vi "Excel Create Printable Sheet.vi"(0 "Sheets Ref In":refnum<k7>, 1 "RowsFirstHeader":i32, 2 "RowsHeadersAfter":i32, 5 "Stat Array":string[][](array[string]), 7 "CMD Step":dbl format="%#_13g", 9 "HeaderInfo":string[](array[string]), 11 "Error In":errorcluster, 12 "RowsFirstPage":i32, 13 "RowsPagesAfter":i32) -> (4 "Sheets Ref Out":refnum<k7>, 15 "Error Out":errorcluster)   [LabVIEW 2013]
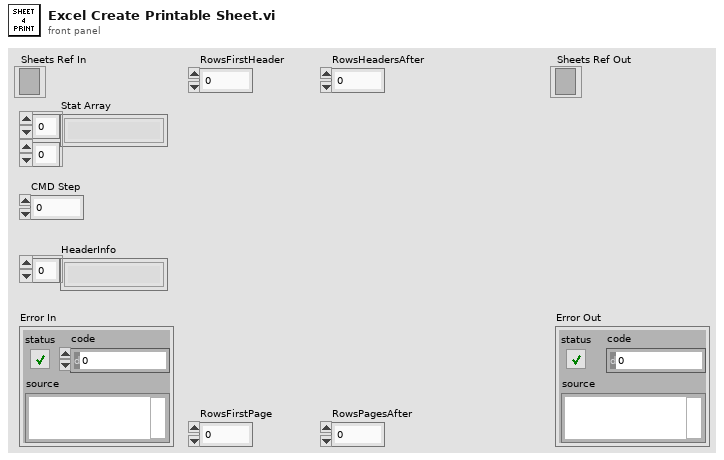
[diagram p1: front panel]
types:
  T1 = cluster{"StartData":i32, "SectionLength":i32, "Have2Split":bool}
  T2 = cluster{"PageStartingIndex":i32, "PageLength":i32}[]
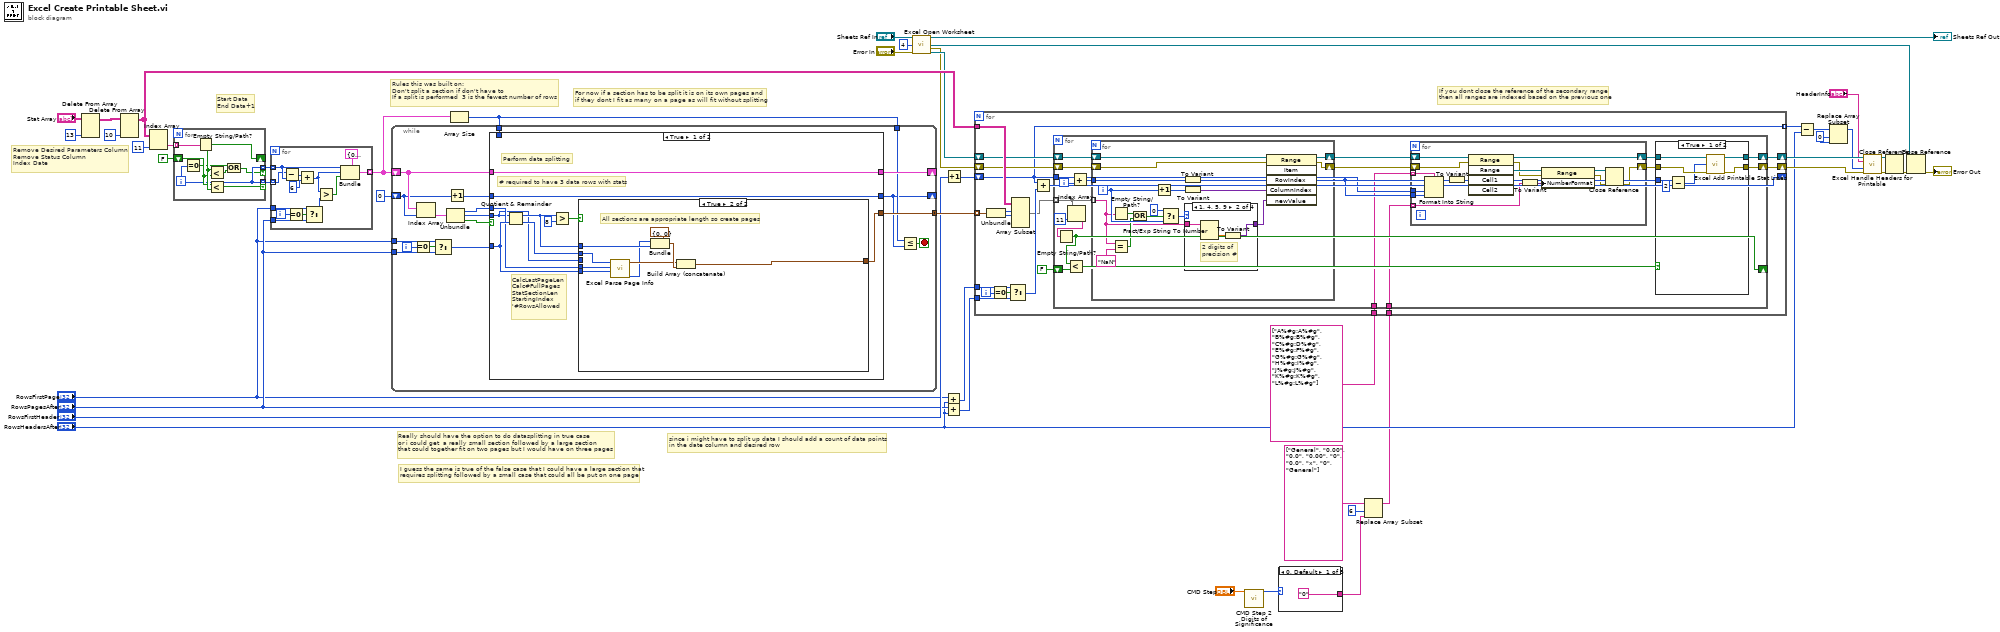
[diagram p0: block diagram]
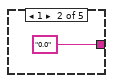
[diagram p2: hidden frame]
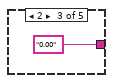
[diagram p3: hidden frame]
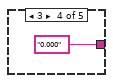
[diagram p4: hidden frame]
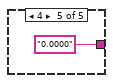
[diagram p5: hidden frame]
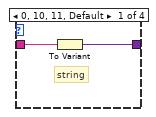
[diagram p7: hidden frame]
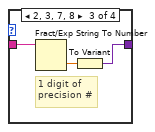
[diagram p8: hidden frame]
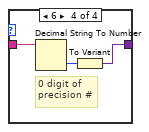
[diagram p9: hidden frame]
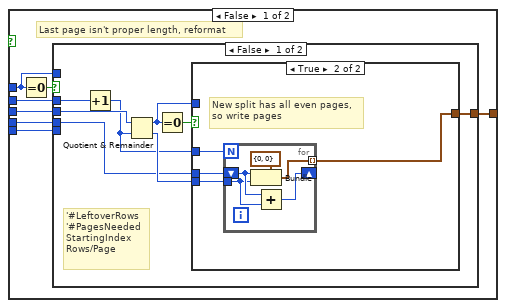
[diagram p10: hidden frame]
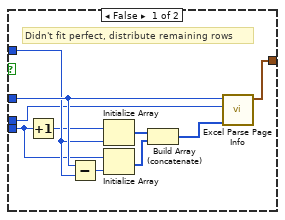
[diagram p11: hidden frame]
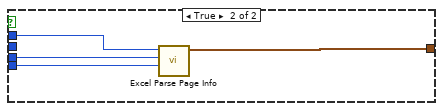
[diagram p12: hidden frame]
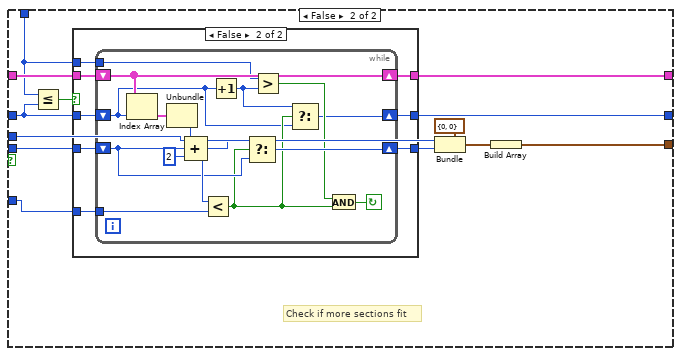
[diagram p13: hidden frame]
diagram:
  w31 = 0 ("index")
  # "If you dont close the reference of the secondary range\nthen all ranges are indexed based on the previous one"
  # "Rules this was built on:\nDon't split a section if don't have to\nIf a split is performed  3 is the fewest number of rows"
  # "For now if a section has to be split it is on its own pages and\nif they dont I fit as many on a page as will fit without splitting"
  # "since i might have to split up data I should add a count of data points\nin the date column and desired row"
  # "I guess the same is true of the false case that I could have a large section that\nrequires splitting followed by a small case that could all be put on one page"
  # "Really should have the option to do datasplitting in true case\nor i could get  a really small section followed by a large section\nthat could together fit on two pages but I would have on three pages"
  # "Start Data\nEnd Data+1"
  # "Remove Desired Parameters Column\nRemove Status Column\nIndex Date"
  n1 = Delete From Array(array="Stat Array", index (col)=13 ("disabled index (col)")) -> (array with subset deleted=w45:string[][])  [unwired: 2 in, 1 out]
  n2 = Delete From Array(array=w45, index (col)=10 ("disabled index (col)")) -> (array with subset deleted=w34:string[][])  [unwired: 2 in, 1 out]
  n3 = Index Array(array=w34, index (col)=11 ("disabled index (col)")) -> (element=w41:string[])  [unwired: 1 in]
  n4 = for {
    tunnel: w41 -> [w54] mode=indexing
    shift-right: [w53] -> _
    shift-left: FALSE -> [w52]
    tunnel: [w50] -> w39 mode=indexing if=w49
    tunnel: [w50] -> w38 mode=indexing if=w51
    i -> [w50]
    n5 = Equal To 0?(x=w50) -> (x = 0?=w47:bool)
    n6 = Empty String/Path?(string/path=w54) -> (empty?=w53:bool)
    n7 = Less?(x=w53, y=w52) -> (x < y?=w48:bool)
    n8 = Less?(x=w52, y=w53) -> (x < y?=w51:bool)
    n9 = Or(x=w47, y=w48) -> (x .or. y?=w49:bool)
  }
  n10 = for {
    tunnel: w39 -> [w67] mode=indexing
    tunnel: w38 -> [w66] mode=indexing
    tunnel: [w65] -> w36 mode=indexing
    tunnel: "RowsFirstPage" -> [w59]
    tunnel: "RowsPagesAfter" -> [w58]
    i -> [w60]
    n11 = Subtract(x=w66, y=w67) -> (x-y=w64:i32)
    n12 = Equal To 0?(x=w60) -> (x = 0?=w61:bool)
    n13 = Add(x=w64, y=6) -> (x+y=w57:i32)
    n14 = Select(t=w59, s=w61, f=w58) -> (s? t:f=w56:i32)
    n15 = Greater?(x=w57, y=w56) -> (0:w55:bool)
    n16 = Bundle(cluster=T1 {"StartData"=0, "SectionLength"=0, "Have2Split"=FALSE}, "StartData"=w67, "SectionLength"=w57, "Have2Split"=w55) -> (w65:T1)
  }
  n17 = Array Size(array=w36) -> (size(s)=w13:i32)
  n18 = while {
    tunnel: "RowsFirstPage" -> [w85]
    tunnel: "RowsPagesAfter" -> [w84]
    shift-right: [w83] -> _
    shift-left: w36 -> [w70]
    shift-right: [w73] -> _
    shift-left: 0 -> [w69]
    tunnel: w13 -> [w74]
    tunnel: [w75] -> w35 mode=concatenating
    tunnel: w13 -> [w71]
    i -> [w77]
    stop <- w72 stop-if-true
    n19 = Equal To 0?(x=w77) -> (x = 0?=w78:bool)
    n20 = Index Array(array=w70, index=w69) -> (element=w68:T1)
    n21 = Select(t=w85, s=w78, f=w84) -> (s? t:f=w79:i32)
    n22 = Unbundle(w68) -> ("StartData"=w82:i32, "SectionLength"=w81:i32, "Have2Split"=w76:bool)
    n23 = Increment(x=w69) -> (x+1=w80:i32)
    n24 = case shown="True" w76 {
      tunnel: w70 -> [w95 w155]
      tunnel: [w95 w154] -> w83
      tunnel: w82 -> [w89 w150]
      tunnel: w81 -> [w86 w153]
      tunnel: w80 -> [w94 w144]
      tunnel: [w87 w147] -> w75
      tunnel: [w94 w146] -> w73
      tunnel: w79 -> [w90 w152]
      tunnel: w71 -> [_ w145]
      frame True {
        # "CalcLastPageLen\nCalc#FullPages\nStatSectionLen\nStartingIndex\n'#RowsAllowed"
        # "# required to have 3 data rows with stats"
        # "Perform data splitting"
        n25 = Quotient & Remainder(x=w86, y=w90) -> (x-y*floor(x/y)=w88:i32, floor(x/y)=w91:i32)
        n26 = Greater?(x=w88, y=8) -> (0:w92:bool)
        n27 = case shown="True" w92 {
          tunnel: w91 -> [w99 w138]
          tunnel: w90 -> [w100 w137]
          tunnel: w89 -> [w101 w135]
          tunnel: w88 -> [w97 w141]
          tunnel: [w98 w139] -> w87
          tunnel: w86 -> [w96 _]
          frame False {
            # "Last page isn't proper length, reformat"
            n28 = Equal To 0?(x=w97) -> (x = 0?=w102:bool)
            n29 = case shown="False" w102 {
              tunnel: w101 -> [w108 w131]
              tunnel: w100 -> [_ w132]
              tunnel: w99 -> [w103 w130]
              tunnel: [w106 w133] -> w98
              tunnel: w97 -> [_ _]
              tunnel: w96 -> [w107 _]
              frame False {
                # "'#LeftoverRows\n'#PagesNeeded\nStartingIndex\nRows/Page"
                n30 = Increment(x=w103) -> (x+1=w104:i32)
                n31 = Quotient & Remainder(x=w107, y=w104) -> (x-y*floor(x/y)=w105:i32, floor(x/y)=w109:i32)
                n32 = Equal To 0?(x=w105) -> (x = 0?=w110:bool)
                n33 = case shown="True" w110 {
                  tunnel: w109 -> [w115 w124]
                  tunnel: w108 -> [w111 w123]
                  tunnel: [w120 w122] -> w106
                  tunnel: w105 -> [w118 _]
                  tunnel: w104 -> [w119 w121]
                  frame False {
                    # "Didn't fit perfect, distribute remaining rows"
                    n34 = Increment(x=w115) -> (x+1=w116:i32)
                    n35 = Subtract(x=w119, y=w118) -> (x-y=w117:i32)
                    n36 = Initialize Array(w116, w118) -> (w114:i32[])
                    n37 = Initialize Array(w115, w117) -> (w113:i32[])
                    n38 = Build Array (concatenate)(w114, w113) -> (w112:i32[])
                    n39 = call "Excel Parse Page Info.vi"("[PageLengths]"=w112, "StartingIndex"=w111, "# of Pages"=w119) -> ("Page Info"=w120:T2)  [unwired: 7 in, 1 out]
                  }
                  frame True {
                    # "New split has all even pages,\nso write pages"
                    n40 = for {
                      N: w121 -> [_]
                      tunnel: w124 -> [w126]
                      shift-right: [w125] -> _
                      shift-left: w123 -> [w127]
                      tunnel: [w128] -> w122 mode=indexing
                      n41 = Bundle(cluster=cluster{"StartPage":i32, "PageLength":i32} {"StartPage"=0, "PageLength"=0}, "StartPage"=w127, "PageLength"=w126) -> (w128:cluster{"StartPage":i32, "PageLength":i32})
                      n42 = Add(x=w127, y=w126) -> (x+y=w125:i32)
                    }
                  }
                }
              }
              frame True {
                n43 = call "Excel Parse Page Info.vi"("PageLength"=w132, "StartingIndex"=w131, "# of Pages"=w130) -> ("Page Info"=w133:T2)  [unwired: 7 in, 1 out]
              }
            }
          }
          frame True {
            # "All sections are appropriate length so create pages"
            n44 = call "Excel Parse Page Info.vi"("PageLength"=w137, "StartingIndex"=w135, "# of Pages"=w138) -> ("IndexOut"=w134:i32, "Page Info"=w136:T2)  [unwired: 7 in]
            n45 = Bundle(cluster=cluster{"StartPage":i32, "PageLength":i32} {"StartPage"=0, "PageLength"=0}, "StartPage"=w134, "PageLength"=w141) -> (w140:cluster{"StartPage":i32, "PageLength":i32})
            n46 = Build Array (concatenate)(w136, w140) -> (w139:cluster{"StartPage":i32, "PageLength":i32}[])
          }
        }
      }
      frame False {
        # "Check if more sections fit"
        n47 = Less Or Equal?(x=w145, y=w144) -> (x <= y?=w143:bool)
        n48 = case shown="False" w143 {
          tunnel: w155 -> [w158 w166]
          tunnel: [w158 w165] -> w154
          tunnel: w153 -> [w156 w164]
          tunnel: w144 -> [w157 w163]
          tunnel: w152 -> [_ w162]
          tunnel: [w156 w161] -> w149
          tunnel: [w157 w160] -> w146
          tunnel: w145 -> [_ w159]
          frame True {
          }
          frame False {
            n49 = while {
              shift-right: [w181] -> w165
              shift-left: w166 -> [w181]
              shift-right: [w174] -> w161
              shift-left: w164 -> [w175]
              tunnel: w162 -> [w177]
              shift-right: [w168] -> w160
              shift-left: w163 -> [w169]
              tunnel: w159 -> [w167]
              stop <- w173 continue-if-true
              n50 = Index Array(array=w181, index=w169) -> (element=w180:T1)
              n51 = Unbundle(w180) -> ("SectionLength"=w179:i32)  [unwired: 2 out]
              n52 = Compound Arithmetic op=ADD(w179, w175, 2 ("value")) -> (w176:i32)
              n53 = Less?(x=w176, y=w177) -> (x < y?=w171:bool)
              n54 = Increment(x=w169) -> (x+1=w170:i32)
              n55 = Select(t=w176, s=w171, f=w175) -> (s? t:f=w174:i32)
              n56 = Greater?(x=w167, y=w170) -> (0:w172:bool)
              n57 = Select(t=w170, s=w171, f=w169) -> (s? t:f=w168:i32)
              n58 = And(x=w172, y=w171) -> (x .and. y?=w173:bool)
            }
          }
        }
        n59 = Bundle(cluster=cluster{"StartPage":i32, "PageLength":i32} {"StartPage"=0, "PageLength"=0}, "StartPage"=w150, "PageLength"=w149) -> (w148:cluster{"StartPage":i32, "PageLength":i32})
        n60 = Build Array(w148) -> (w147:cluster{"StartPage":i32, "PageLength":i32}[])
      }
    }
    n61 = Less Or Equal?(x=w74, y=w73) -> (x <= y?=w72:bool)
  }
  n62 = call "Excel Open Worksheet.vi"("Sheets Ref In"="Sheets Ref In", "Sheet#"=4, "Error In"="Error In") -> ("Sheets Ref Out"=→"Sheets Ref Out":refnum<k7>, "Worksheet Ref Out"=w21:refnum<k7>, "Error Out"=w28:errorcluster, "Cells Ref Out"=w29:refnum<k7>)  [unwired: 9 in]
  n63 = Add(x="RowsFirstPage", y="RowsHeadersAfter") -> (x+y=w8:i32)
  n64 = Add(x="RowsPagesAfter", y="RowsHeadersAfter") -> (x+y=w11:i32)
  n65 = Increment(x="RowsFirstHeader") -> (x+1=w14:i32)
  n66 = call "CMD Step 2 Digits of Significance.vi"("CMD Step"="CMD Step") -> ("Digits of Significance"=w5:i32)  [unwired: 14 in]
  n67 = case shown="0, Default" w5 {
    tunnel: ["0" "0.0" "0.00" "0.000" "0.0000"] -> w7
    frame 0, Default {
    }
    frame 1 {
    }
    frame 2 {
    }
    frame 3 {
    }
    frame 4 {
    }
  }
  n68 = Replace Array Subset(array=string[] ["General", "0.00", "0.0", "0.00", "0", "0.0", "x", "0", "General"], new element=w7, index=6) -> (w1:string[])
  n69 = for {
    tunnel: w35 -> [w205] mode=indexing
    tunnel: w34 -> [w204]
    shift-right: [w191] -> w27
    shift-left: w29 -> [w201]
    shift-right: [w192] -> w26
    shift-left: w28 -> [w200]
    shift-right: [w196] -> _
    shift-left: w14 -> [w190]
    tunnel: w11 -> [w195]
    tunnel: w8 -> [w194]
    tunnel: [w190] -> w33 mode=indexing
    tunnel: string[] ["A%#g:A%#g", "B%#g:B%#g", "C%#g:D%#g", "E%#g:F%#g", "G%#g:G%#g", "H%#g:I%#g", "J%#g:J%#g", "K%#g:K%#g", "L%#g:L%#g"] -> [w188]
    tunnel: w1 -> [w187]
    i -> [w198]
    n70 = Unbundle(w205) -> ("StartPage"=w203:i32, "PageLength"=w202:i32)
    n71 = Equal To 0?(x=w198) -> (x = 0?=w199:bool)
    n72 = Select(t=w194, s=w199, f=w195) -> (s? t:f=w197:i32)
    n73 = Array Subset(array=w204, index (row)=w203, length (row)=w202) -> (w193:string[][])  [unwired: 2 in]
    n74 = Add(x=w190, y=w197) -> (x+y=w196:i32)
    n75 = for {
      shift-right: [w214] -> w191
      shift-left: w201 -> [w224]
      shift-right: [w215] -> w192
      shift-left: w200 -> [w223]
      tunnel: w193 -> [w221] mode=indexing
      tunnel: w190 -> [w208]
      shift-right: [w218] -> _
      shift-left: FALSE -> [w217]
      tunnel: w188 -> [w207]
      tunnel: w187 -> [w206]
      i -> [w222]
      n76 = Index Array(array=w221, index=11) -> (element=w219:string)
      n77 = Empty String/Path?(string/path=w219) -> (empty?=w218:bool)
      n78 = Less?(x=w218, y=w217) -> (x < y?=w216:bool)
      n79 = Add(x=w208, y=w222) -> (x+y=w209:i32)
      n80 = for {
        shift-right: [w264] -> w213
        shift-left: w224 -> [w265]
        shift-right: [w263] -> w212
        shift-left: w223 -> [w262]
        tunnel: w221 -> [w251] mode=indexing
        tunnel: w209 -> [w254]
        i -> [w257]
        n81 = Empty String/Path?(string/path=w251) -> (empty?=w250:bool)
        n82 = Equal?(x=w251, y="NaN") -> (x = y?=w253:bool)
        n83 = Or(x=w250, y=w253) -> (x .or. y?=w249:bool)
        n84 = Increment(x=w257) -> (x+1=w259:i32)
        n85 = Select(t=0, s=w249, f=w257) -> (s? t:f=w255:i32)
        n86 = To Variant(anything=w254) -> (Variant=w261:variant)
        n87 = To Variant(anything=w259) -> (Variant=w260:variant)
        n88 = case shown="1, 4, 5, 9" w255 {
          tunnel: w251 -> [w267 w270 w273 w276]
          tunnel: [w266 w268 w271 w274] -> w258
          frame 0, 10, 11, Default {
            # "string"
            n89 = To Variant(anything=w267) -> (Variant=w266:variant)
          }
          frame 1, 4, 5, 9 {
            # "2 digits of\nprecision #"
            n90 = Fract/Exp String To Number(string=w270) -> (number=w269:dbl)  [unwired: 3 in, 1 out]
            n91 = To Variant(anything=w269) -> (Variant=w268:variant)
          }
          frame 2, 3, 7, 8 {
            # "1 digit of\nprecision #"
            n92 = Fract/Exp String To Number(string=w273) -> (number=w272:dbl)  [unwired: 3 in, 1 out]
            n93 = To Variant(anything=w272) -> (Variant=w271:variant)
          }
          frame 6 {
            # "0 digit of\nprecision #"
            n94 = Decimal String To Number(string=w276) -> (number=w275:i32)  [unwired: 2 in, 1 out]
            n95 = To Variant(anything=w275) -> (Variant=w274:variant)
          }
        }
        n96 = invoke class="Range" method="Item"(reference=w265, error in=w262, "RowIndex"=w261, "ColumnIndex"=w260, "newValue"=w258) -> (reference out=w264:refnum<k7>, error out=w263:errorcluster)  [unwired: 1 in, 4 out]
      }
      n97 = for {
        shift-right: [w227] -> w211
        shift-left: w213 -> [w233]
        shift-right: [w226] -> w210
        shift-left: w212 -> [w232]
        tunnel: w206 -> [w237] mode=indexing
        tunnel: w207 -> [w236] mode=indexing
        tunnel: w208 -> [w235]
        tunnel: w209 -> [w225]
        n98 = Format Into String(format string=w236, w235, w225) -> (resulting string=w239:string)  [unwired: 2 in, 1 out]
        n99 = To Variant(anything=w239) -> (Variant=w234:variant)
        n100 = invoke class="Range" method="Range"(reference=w233, error in=w232, "Cell1"=w234) -> (reference out=w227:refnum<k7>, error out=w230:errorcluster, "Range"=w231:refnum<k7>)  [unwired: 2 in, 2 out]
        n101 = To Variant(anything=w237) -> (Variant=w238:variant)
        n102 = property class="Range"(reference=w231, error in=w230, "NumberFormat"=w238) -> (reference out=w229:refnum<k7>, error out=w228:errorcluster)
        n103 = Close Reference(reference=w229, error in (no error)=w228) -> (error out=w226:errorcluster)
      }
      n104 = case shown="True" w216 {
        tunnel: w210 -> [w244 w247]
        tunnel: w211 -> [w243 w248]
        tunnel: [w242 w247] -> w215
        tunnel: [w241 w248] -> w214
        tunnel: w209 -> [w246 _]
        frame True {
          n105 = Subtract(x=w246, y=2) -> (x-y=w240:i32)
          n106 = call "Excel Add Printable Stat Lines.vi"("CellsRefIn"=w243, "RowIndex"=w240, "ErrorIn"=w244) -> ("CellsRefOut"=w241:refnum<k7>, "ErrorOut"=w242:errorcluster)  [unwired: 11 in]
        }
        frame False {
        }
      }
    }
  }
  n107 = Subtract(x=w33, y="RowsHeadersAfter") -> (x-y=w32:i32[])
  n108 = Replace Array Subset(array=w32, new element=w31, index=w31) -> (w25:i32[])
  n109 = call "Excel Handle Headers for Printable.vi"("CellsRefIn"=w27, "HeaderInfo"="HeaderInfo", "IndexesPageStart"=w25, "ErrorIn"=w26) -> ("RefCellsOut"=w22:refnum<k7>, "ErrorOut"=w23:errorcluster)  [unwired: 10 in]
  n110 = Close Reference(reference=w22, error in (no error)=w23) -> (error out=w20:errorcluster)
  n111 = Close Reference(reference=w21, error in (no error)=w20) -> (error out=→"Error Out":errorcluster)
